vi "_Main_ByRuns_DAC2022_V1.1.0.vi"() -> ()   [LabVIEW 2017]
uses:
  <vilib>/Instr/_visa.llb/VISA Configure Serial Port (Instr).vi
panel:
  in  "Bias, kV/cm":dbl
  out "Field, kV/cm":dbl
  out "Current, mA":dbl
  out "Voltage, V":dbl
  in  "WaveForm":i32(listbox)
  in  "Auto\nturn OFF":bool=TRUE
  in  "Content":i32(listbox)
  out "LastTrigTimer, s":dbl
  in  "Graph every, cycle":dbl=10.0 min=1.0 max=100.0
  in  "SendPeriod, ms":dbl=100.0 min=10.0 max=10000.0
  out "RunsNeed":i32
  out "Time LOG":cluster{dbl[], dbl[]}(graph)
  out "TrigTimer, s":dbl
  out "Bytes at Port":u32
  out "RecTry":i32
  in  "Exposition, s":dbl=3.0
  out "Channel 2, V":dbl format="%#_5g"
  out "Channel 1, V":dbl format="%#_5g"
  in  "Stop Button":bool
  in  "Start Button":bool
  in  "Sample H, um":dbl=32.0
  out "VoltageArray, V":dbl[](array[numeric])
  out "Shutter Red":bool
  out "Shutter Green":bool
  in  "Frames In Run":u32=180
  out "Global Frame Done":u32
  out "Now is Run #":u32
  out "Frame In Run Done":u32
  in  "Step, kV/cm":dbl=1.0 min=0.01 max=1000.0
  in  "Amplitude, kV/cm":dbl=10.0 min=10.0 max=1500.0
  in  "LOG file":path
  in  "COM ADC":refnum<visa-resource-name>
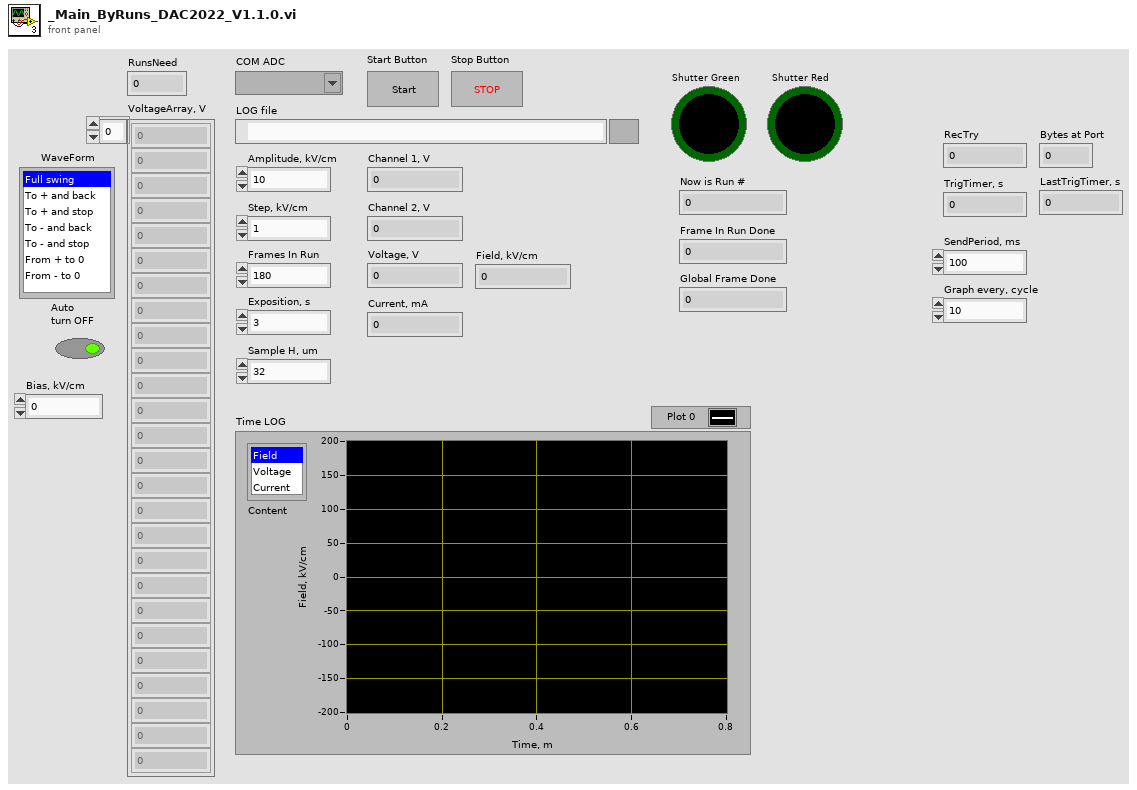
[diagram p1: front panel]
types:
  T1 = cluster{i32, i32, u32, "TrigState":bool, "TrigTimer, s":dbl, "CurrentError":bool}
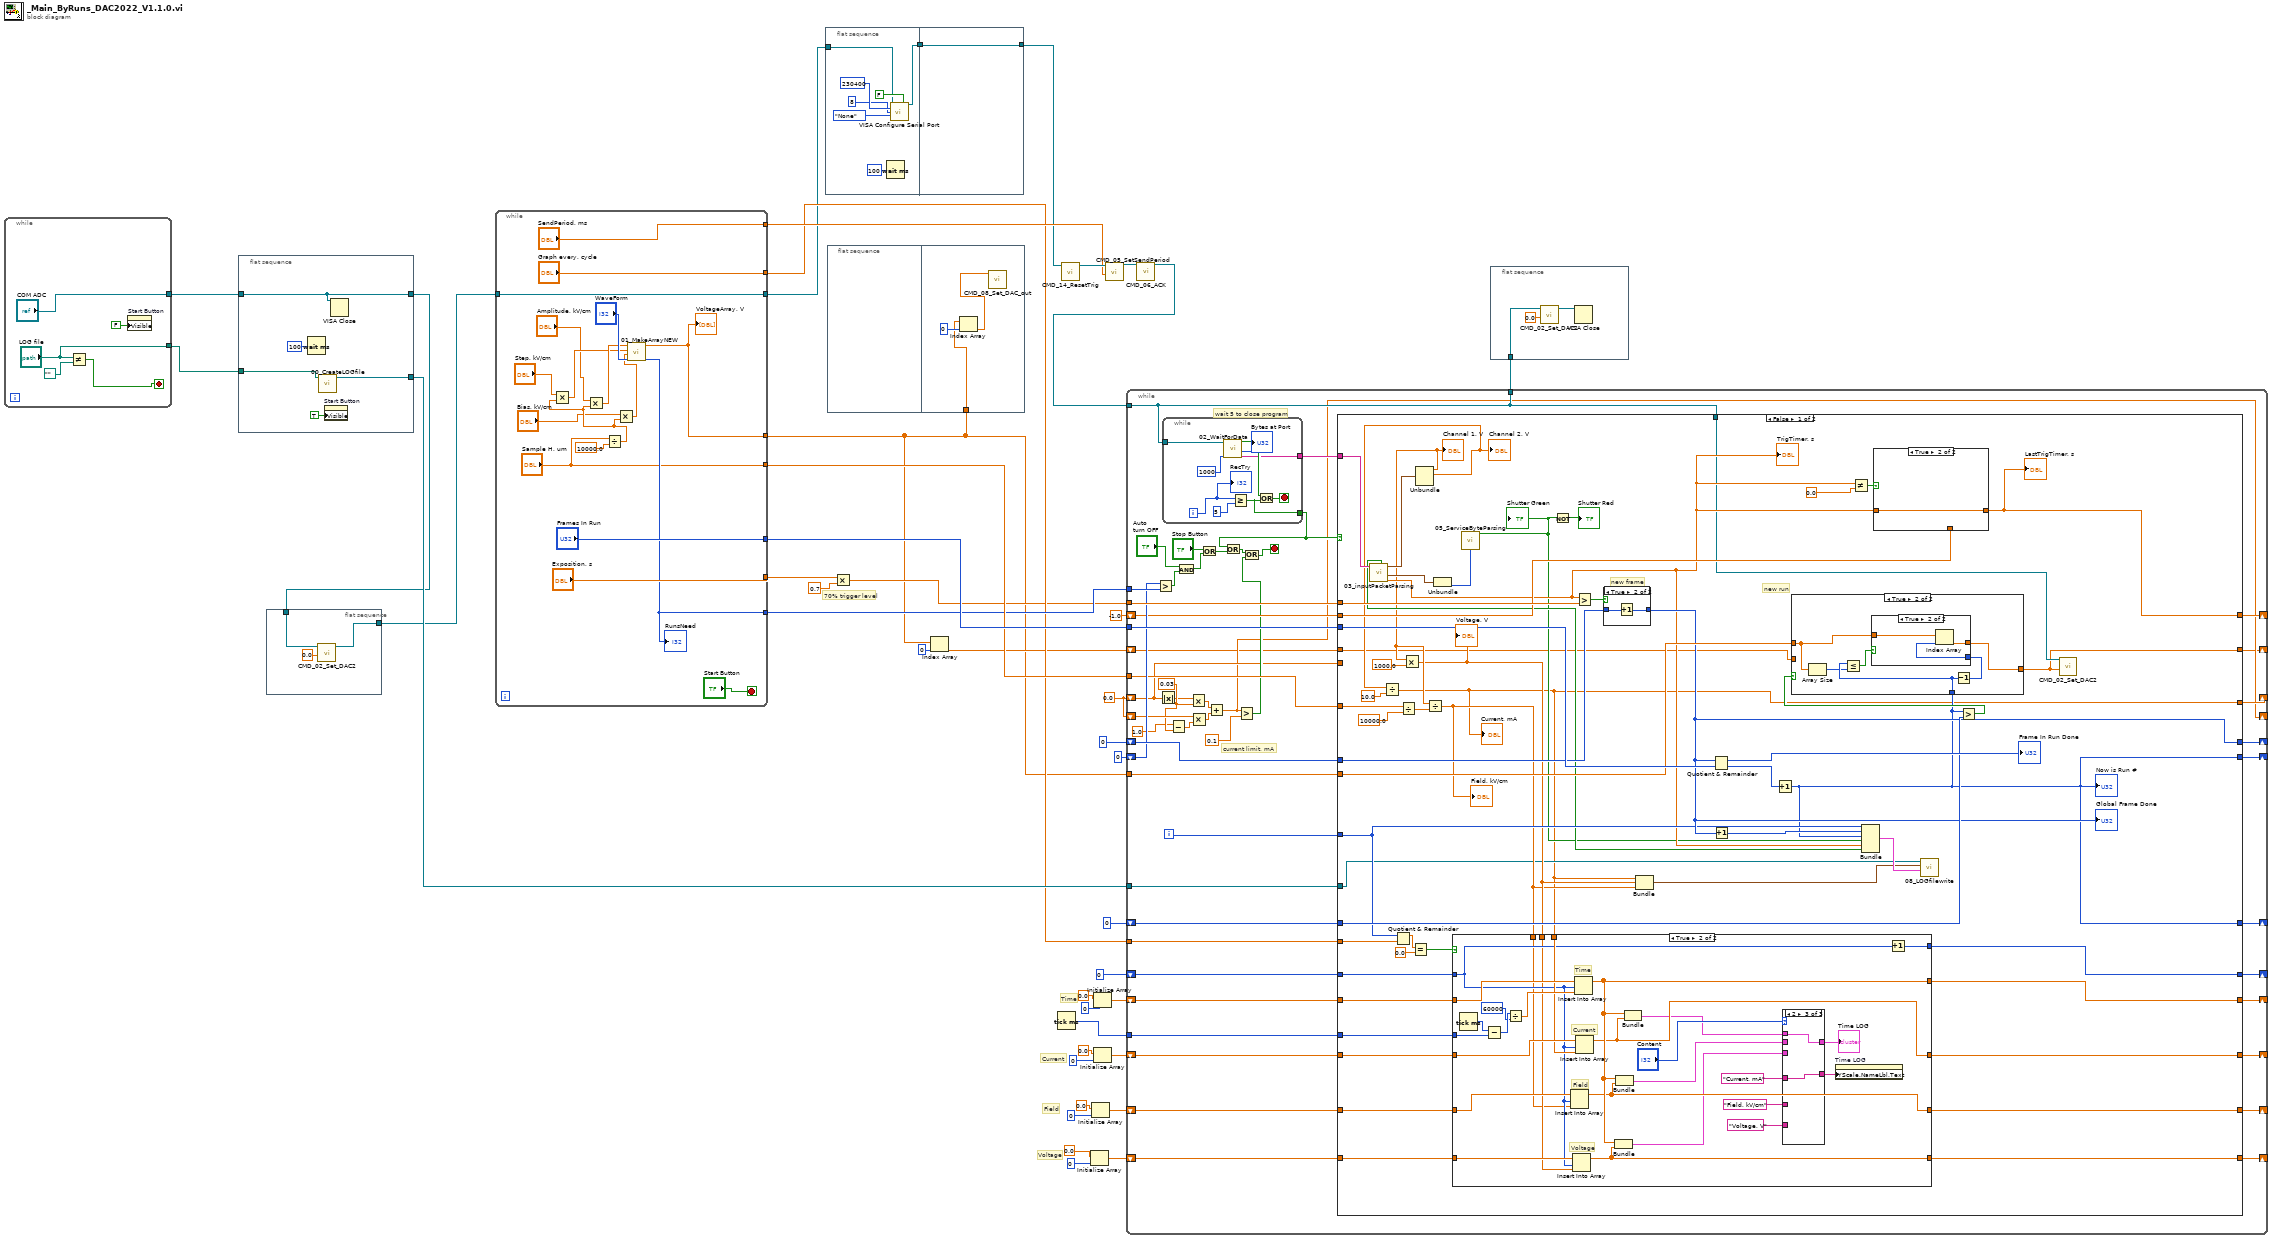
[diagram p0: block diagram]
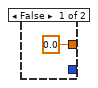
[diagram p7: hidden frame]
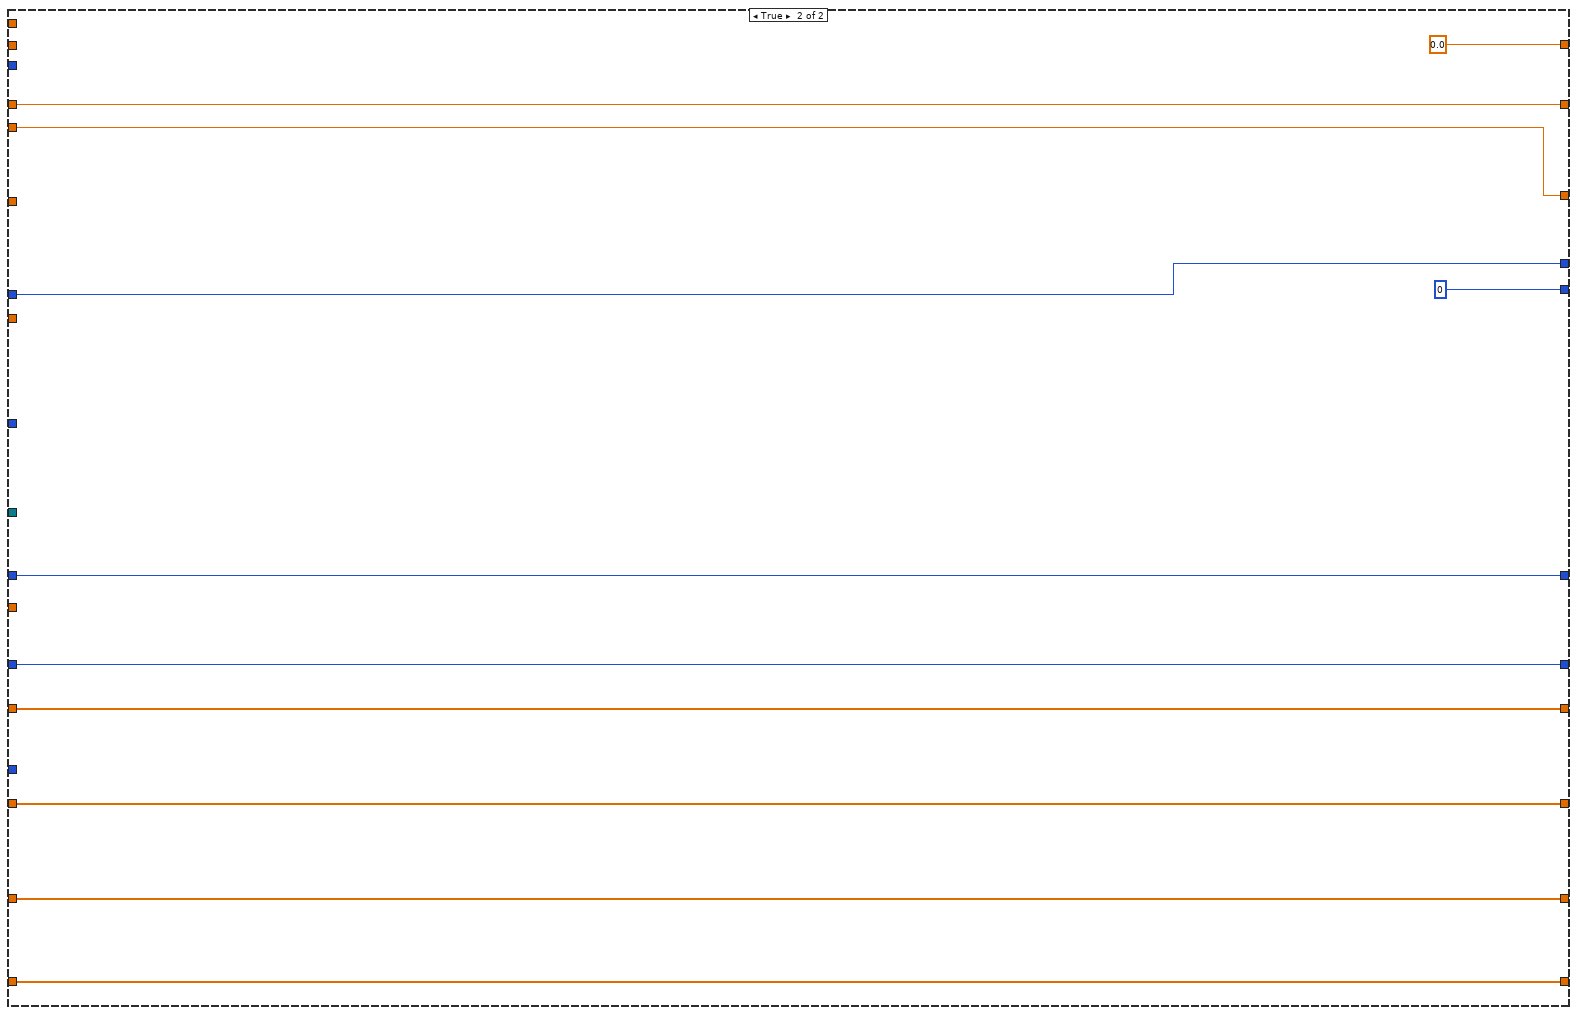
[diagram p9: hidden frame]
diagram:
  w6 = 0.0
  # "70% trigger level"
  # "Voltage"
  # "Field"
  # "Time"
  # "Current"
  n1 = while {
    tunnel: ["COM ADC"] -> w12
    tunnel: ["LOG file"] -> w11
    stop <- w43 stop-if-true
    n2 = Not Equal?(x="LOG file", y=path "" ("LOG file")) -> (x != y?=w43:bool)
    n3 = property on="Start Button" class="Bool"("Visible"=FALSE) -> ()  [unwired: 2 in, 2 out]
  }
  n4 = flat-sequence {
    tunnel: [w52] -> w40
    tunnel: w12 -> [w48]
    tunnel: w11 -> [w49]
    tunnel: [w48] -> w5
    frame #0 {
      n5 = Wait (ms)(milliseconds to wait=u32 100) -> ()  [unwired: 1 out]
      n6 = call "00_CreateLOGfile.vi"("LOG file"=w49) -> ("refnum out"=w52:refnum<file>)  [unwired: 10 in]
      n7 = property on="Start Button" class="Bool"("Visible"=TRUE) -> ()  [unwired: 2 in, 2 out]
      n8 = VISA Close(VISA resource name=w48) -> ()  [unwired: 1 in, 1 out]
    }
  }
  n9 = flat-sequence {
    tunnel: w5 -> [w55]
    tunnel: [w54] -> w4
    frame #0 {
      n10 = call "CMD_02_Set_DAC2.vi"("Input, V"=0.0, "VISA resource name"=w55) -> ("VISA resource name out"=w54:refnum<visa-resource-name>)  [unwired: 9 in]
    }
  }
  n11 = while {
    tunnel: w4 -> [w67]
    tunnel: [w67] -> w9
    tunnel: [w66] -> w1
    tunnel: ["Sample H, um"] -> w41
    tunnel: ["Frames In Run"] -> w42
    tunnel: ["Exposition, s"] -> w21
    tunnel: [w65] -> w26
    tunnel: ["SendPeriod, ms"] -> w24
    tunnel: ["Graph every, cycle"] -> w23
    stop <- "Start Button" stop-if-true
    n12 = Divide(x="Sample H, um", y=10000.0) -> (x/y=w58:dbl)
    n13 = Multiply(x="Step, kV/cm", y=w58) -> (x*y=w61:dbl)
    n14 = Multiply(x="Amplitude, kV/cm", y=w58) -> (x*y=w62:dbl)
    n15 = Multiply(x="Bias, kV/cm", y=w58) -> (x*y=w56:dbl)
    n16 = call "01_MakeArrayNEW.vi"("Amp"=w62, "Step"=w61, "Bias"=w56, "WaveForm"="WaveForm") -> ("Array"=w66:dbl[], "ArraySize"=w65:i32)  [unwired: 5 in]
    "VoltageArray, V" <- w66
    "RunsNeed" <- w65
  }
  n17 = flat-sequence {
    tunnel: w9 -> [w76]
    tunnel: [w75] -> w10
    tunnel: w10 -> [w81]
    tunnel: [w81] -> w8
    frame #0 {
      n18 = Wait (ms)(milliseconds to wait=u32 100) -> ()  [unwired: 1 out]
      n19 = call-poly "VISA Configure Serial Port"("VISA resource name"=w76, "Enable Termination\nChar (T)"=FALSE ("Enable Termination\nChar (T)"), "baud rate (9600)"=u32 230400, "data bits (8)"=u16 8, "parity (0:none)"=enum16{"None", "Odd", "Even", "Mark", "Space"}."None") -> ("VISA resource name out"=w75:refnum<visa-resource-name>)  [unwired: 9 in, 1 out]
    }
    frame #1 {
    }
  }
  n20 = flat-sequence {
    tunnel: w1 -> [w83]
    frame #0 {
    }
    frame #1 {
      n21 = Index Array(array=w83, index=0) -> (element=w82:dbl)
      n22 = call "CMD_08_Set_DAC_out.vi"("DAC voltage, V"=w82) -> ()  [unwired: 11 in]
    }
  }
  n23 = Multiply(x=w21, y=0.7) -> (x*y=w22:dbl)
  n24 = Index Array(array=w1, index=0) -> (element=w3:dbl)
  n25 = Tick Count (ms)() -> (millisecond timer value=w30:u32)
  n26 = call "CMD_14_ResetTrig.vi"("VISA resource name"=w8) -> ("VISA resource name out"=w37:refnum<visa-resource-name>)  [unwired: 10 in]
  n27 = Initialize Array(0.0 ("element"), 0 ("dimension size")) -> (w13:dbl[])
  n28 = Initialize Array(0.0 ("element"), 0 ("dimension size")) -> (w14:dbl[])
  n29 = Initialize Array(0.0 ("element"), 0 ("dimension size")) -> (w27:dbl[])
  n30 = Initialize Array(0.0 ("element"), 0 ("dimension size")) -> (w31:dbl[])
  n31 = call "CMD_05_SetSendPeriod.vi"("Period, ms"=w24, "VISA resource name"=w37) -> ("VISA resource name out"=w36:refnum<visa-resource-name>)  [unwired: 9 in]
  n32 = call "CMD_06_ACK.vi"("VISA resource name"=w36) -> ("VISA resource name out"=w35:refnum<visa-resource-name>)  [unwired: 10 in]
  n33 = while {
    tunnel: w35 -> [w102]
    tunnel: w1 -> [w125]
    tunnel: w42 -> [w131]
    tunnel: w22 -> [w133]
    tunnel: w41 -> [w103]
    tunnel: w40 -> [w132]
    shift-right: [w128] -> _
    shift-left: 0 -> [w130]
    shift-right: [w127] -> _
    shift-left: u32 0 -> [w126]
    shift-right: [w123] -> _
    shift-left: 0 -> [w124]
    tunnel: w30 -> [w121]
    shift-right: [w119] -> _
    shift-left: w31 -> [w122]
    shift-right: [w118] -> _
    shift-left: w27 -> [w120]
    tunnel: w26 -> [w114]
    shift-right: [w116] -> _
    shift-left: u32 0 -> [w113]
    tunnel: w23 -> [w110]
    shift-right: [w109] -> _
    shift-left: -1.0 ("TrigTimer, s") -> [w108]
    shift-right: [w105] -> _
    shift-left: w14 -> [w107]
    shift-right: [w104] -> _
    shift-left: w13 -> [w106]
    tunnel: [w102] -> w7
    shift-right: [w101] -> _
    shift-left: w6 -> [w96]
    shift-right: [w87] -> _
    shift-left: w6 -> [w95]
    shift-right: [w86] -> _
    shift-left: w3 -> [w85]
    i -> [w129]
    stop <- w99 stop-if-true
    w93 = 0.03
    # "current limit, mA"
    # "wait 5 to close program"
    n34 = Greater?(x=w113, y=w114) -> (0:w111:bool)
    n35 = Absolute Value(x=w96) -> (abs(x)=w88:dbl)
    n36 = while {
      tunnel: w102 -> [w257]
      tunnel: [w260] -> w135
      tunnel: [w261] -> w134
      i -> [w259]
      stop <- w263 stop-if-true
      n37 = call "02_WaitForData.vi"("WaitTimeoutMS"=u32 1000, "VISA"=w257) -> ("Buffer"=w261:string, "Bytes at Port"=→"Bytes at Port":u32, "Data Recived"=w262:bool)  [unwired: 7 in]
      n38 = Greater Or Equal?(x=w259, y=5) -> (x >= y?=w260:bool)
      n39 = Or(x=w262, y=w260) -> (x .or. y?=w263:bool)
      "RecTry" <- w259
    }
    n40 = Subtract(x=1.0, y=w93) -> (x-y=w94:dbl)
    n41 = And(x="Auto\nturn OFF", y=w111) -> (x .and. y?=w112:bool)
    n42 = Multiply(x=w88, y=w93) -> (x*y=w90:dbl)
    n43 = Multiply(x=w95, y=w94) -> (x*y=w91:dbl)
    n44 = Or(x="Stop Button", y=w112) -> (x .or. y?=w117:bool)
    n45 = Add(x=w90, y=w91) -> (x+y=w87:dbl)
    n46 = Or(x=w135, y=w117) -> (x .or. y?=w98:bool)
    n47 = Greater?(x=w87, y=0.1) -> (0:w97:bool)
    n48 = Or(x=w98, y=w97) -> (x .or. y?=w99:bool)
    n49 = case shown="False" w135 {
      tunnel: w134 -> [w191 _]
      tunnel: w133 -> [w187 _]
      tunnel: w132 -> [w140 _]
      tunnel: w131 -> [w188 _]
      tunnel: w130 -> [w185 w256]
      tunnel: w129 -> [w173 _]
      tunnel: [w178 w256] -> w128
      tunnel: [w164 w255] -> w127
      tunnel: w126 -> [w180 w255]
      tunnel: w125 -> [w181 _]
      tunnel: w102 -> [w138 _]
      tunnel: w124 -> [w171 w254]
      tunnel: [w170 w254] -> w123
      tunnel: w122 -> [w169 w253]
      tunnel: w121 -> [w168 _]
      tunnel: w120 -> [w167 w252]
      tunnel: [w166 w253] -> w119
      tunnel: [w165 w252] -> w118
      tunnel: [w164 u32 0] -> w116
      tunnel: w110 -> [w163 _]
      tunnel: [w160 0.0 ("TrigTimer, s")] -> w109
      tunnel: w108 -> [w159 _]
      tunnel: w107 -> [w155 w249]
      tunnel: w106 -> [w154 w248]
      tunnel: [w153 w249] -> w105
      tunnel: [w152 w248] -> w104
      tunnel: w103 -> [w146 _]
      tunnel: [w139 w247] -> w101
      tunnel: w96 -> [_ w247]
      tunnel: [w137 w246] -> w86
      tunnel: w85 -> [w136 w246]
      frame False {
        # "new run"
        # "new frame"
        n50 = call "03_inputPacketParsing.vi"("string"=w191) -> ("TrigTimer, s"=w158:dbl, "Service state"=w177:cluster{u8, u8}, "Voltage"=w189:cluster{dbl, dbl, dbl, dbl}, "CurrentError"=w157:bool)  [unwired: 6 in, 1 out]
        "TrigTimer, s" <- w158
        n51 = Quotient & Remainder(x=w173, y=w163) -> (x-y*floor(x/y)=w175:dbl)  [unwired: 1 out]
        n52 = Divide(x=w146, y=10000.0) -> (x/y=w147:dbl)
        n53 = Equal?(x=w175, y=0.0) -> (x = y?=w172:bool)
        n54 = Unbundle(w189) -> (w148:dbl, w150:dbl)  [unwired: 2 out]
        "Channel 1, V" <- w148
        "Channel 2, V" <- w150
        n55 = Divide(x=w150, y=10.0) -> (x/y=w139:dbl)
        "Current, mA" <- w139
        n56 = Multiply(x=w148, y=1000.0) -> (x*y=w143:dbl)
        "Voltage, V" <- w143
        n57 = Divide(x=w148, y=w147) -> (x/y=w142:dbl)
        "Field, kV/cm" <- w142
        n58 = Unbundle(w177) -> (w176:u8)  [unwired: 1 out]
        n59 = case shown="True" w172 {
          tunnel: w171 -> [w198 w214]
          tunnel: [w198 w221] -> w170
          tunnel: w169 -> [w196 w219]
          tunnel: w168 -> [_ w224]
          tunnel: w167 -> [w197 w218]
          tunnel: [w197 w210] -> w165
          tunnel: [w196 w213] -> w166
          tunnel: w139 -> [_ w217]
          tunnel: w155 -> [w195 w216]
          tunnel: w154 -> [w194 w215]
          tunnel: [w195 w211] -> w153
          tunnel: [w194 w212] -> w152
          tunnel: w143 -> [_ w200]
          tunnel: w142 -> [_ w199]
          frame False {
          }
          frame True {
            # "Time"
            # "Voltage"
            # "Field"
            # "Current"
            n60 = Tick Count (ms)() -> (millisecond timer value=w225:u32)
            n61 = Subtract(x=w225, y=w224) -> (x-y=w223:u32)
            n62 = Divide(x=w223, y=u32 60000) -> (x/y=w220:dbl)
            n63 = Insert Into Array(array=w216, index=w214, new element=w199) -> (w211:dbl[])
            n64 = Insert Into Array(array=w215, index=w214, new element=w200) -> (w212:dbl[])
            n65 = Insert Into Array(array=w219, index=w214, new element=w220) -> (w213:dbl[])
            n66 = Insert Into Array(array=w218, index=w214, new element=w217) -> (w210:dbl[])
            n67 = Bundle(w213, w212) -> (w206:cluster{dbl[], dbl[]})  [unwired: 1 in]
            n68 = Bundle(w213, w211) -> (w207:cluster{dbl[], dbl[]})  [unwired: 1 in]
            n69 = Bundle(w213, w210) -> (w208:cluster{dbl[], dbl[]})  [unwired: 1 in]
            n70 = case shown="2" "Content" {
              tunnel: w208 -> [_ _ w231]
              tunnel: w207 -> [w227 _ _]
              tunnel: w206 -> [_ w229 _]
              tunnel: [w227 w229 w231] -> w205
              tunnel: "Current, mA" ("Y Scale.Name Label.Text") -> [_ _ w230]
              tunnel: "Field, kV/cm" ("Y Scale.Name Label.Text") -> [w226 _ _]
              tunnel: "Voltage, V" ("Y Scale.Name Label.Text") -> [_ w228 _]
              tunnel: [w226 w228 w230] -> w201
              frame 0, Default {
              }
              frame 1 {
              }
              frame 2 {
              }
            }
            "Time LOG" <- w205
            n71 = property on="Time LOG" class="XYGraph (strict)"("YScale.NameLbl.Text"=w201) -> ()  [unwired: 2 in, 2 out]
            n72 = Increment(x=w214) -> (x+1=w221:i32)
          }
        }
        n73 = call "05_ServiceByteParsing.vi"("InputByte"=w176) -> ("TrigState"=w156:bool)  [unwired: 7 in, 3 out]
        "Shutter Green" <- w156
        n74 = Not(x=w156) -> (.not. x?=→"Shutter Red":bool)
        n75 = Greater?(x=w158, y=w187) -> (0:w186:bool)
        n76 = case shown="True" w186 {
          tunnel: w185 -> [w243 w245]
          tunnel: [w243 w244] -> w178
          frame False {
          }
          frame True {
            n77 = Increment(x=w245) -> (x+1=w244:i32)
          }
        }
        "Global Frame Done" <- w178
        n78 = Bundle(w139, w143, w142) -> (w141:cluster{dbl, dbl, dbl})  [unwired: 1 in]
        n79 = Quotient & Remainder(x=w178, y=w188) -> (x-y*floor(x/y)=→"Frame In Run Done":u32, floor(x/y)=w183:u32)
        n80 = Increment(x=w178) -> (x+1=w179:i32)
        n81 = Increment(x=w183) -> (x+1=w164:u32)
        "Now is Run #" <- w164
        n82 = Not Equal?(x=w158, y=0.0) -> (x != y?=w162:bool)
        n83 = Bundle(w173, w179, w164, "TrigState"=w156, "TrigTimer, s"=w158, "CurrentError"=w157) -> (w144:T1)  [unwired: 1 in]
        n84 = case shown="True" w162 {
          tunnel: [w192 w193] -> w160
          tunnel: w158 -> [_ w193]
          tunnel: w159 -> [w192 _]
          frame False {
          }
          frame True {
          }
        }
        "LastTrigTimer, s" <- w160
        n85 = call "08_LOGfilewrite.vi"("Counters"=w144, "output cluster"=w141, "refnum out"=w140) -> ()  [unwired: 9 in]
        n86 = Greater?(x=w164, y=w180) -> (0:w184:bool)
        n87 = case shown="True" w184 {
          tunnel: w181 -> [_ w234]
          tunnel: w164 -> [_ w237]
          tunnel: [w232 w233] -> w137
          tunnel: w136 -> [w232 _]
          frame False {
          }
          frame True {
            n88 = Array Size(array=w234) -> (size(s)=w236:i32)
            n89 = Less Or Equal?(x=w237, y=w236) -> (x <= y?=w235:bool)
            n90 = Decrement(x=w237) -> (x-1=w238:u32)
            n91 = case shown="True" w235 {
              tunnel: w238 -> [_ w242]
              tunnel: w234 -> [_ w241]
              tunnel: [0.0 w240] -> w233
              frame False {
              }
              frame True {
                n92 = Index Array(array=w241, index=w242) -> (element=w240:dbl)
              }
            }
          }
        }
        n93 = call "CMD_02_Set_DAC2.vi"("Input, V"=w137, "VISA resource name"=w138) -> ()  [unwired: 9 in, 1 out]
      }
      frame True {
      }
    }
  }
  n94 = flat-sequence {
    tunnel: w7 -> [w267]
    frame #0 {
      n95 = call "CMD_02_Set_DAC2.vi"("Input, V"=0.0, "VISA resource name"=w267) -> ("VISA resource name out"=w266:refnum<visa-resource-name>)  [unwired: 9 in]
      n96 = VISA Close(VISA resource name=w266) -> ()  [unwired: 1 in, 1 out]
    }
  }
